vi "ADQ214 Get Afe Switch.vi"(7 "afe":string, 8 "error in (no error)":errorcluster, 9 "channel":u8, 10 "adq214_num":i32, 11 "adq_cu_ptr":u32) -> (0 "error out":errorcluster, 2 "function return":u32, 3 "adq_cu_ptr out":u32, 5 "afe out":string)   [LabVIEW 8.6, in "ADQAPI.lvlib"]
doc: "extern \"C\" __declspec(dllimport) unsigned int ADQ214_GetAfeSwitch(void* adq_cu_ptr, int adq214_num, unsigned char channel, unsigned char* afe);"
uses:
  F/HRT/Sp Devices Thesis/ADQ-214 project (H R)/ADQAPI.lvlib
  F:/HRT/Sp Devices Thesis/ADQ-214 project (H R)/ADQAPI.dll
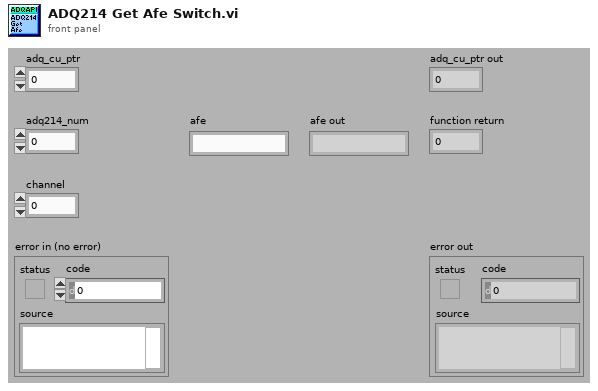
[diagram p1: front panel]
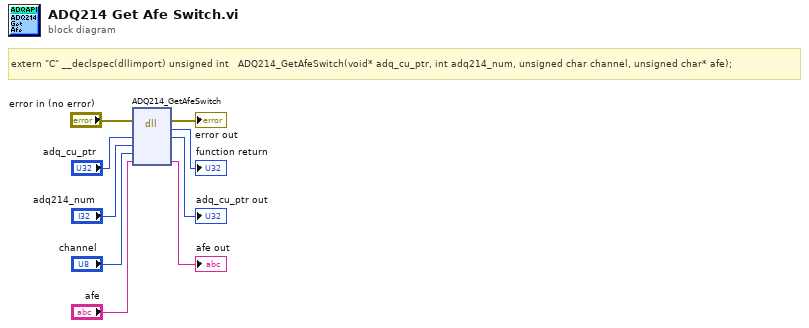
[diagram p0: block diagram]
diagram:
  # "extern \"C\" __declspec(dllimport) unsigned int   ADQ214_GetAfeSwitch(void* adq_cu_ptr, int adq214_num, unsigned char channel, unsigned char* afe);"
  n1 = dll-call lib="F:/HRT/Sp Devices Thesis/ADQ-214 project (H R)/ADQAPI.*" fn="ADQ214_GetAfeSwitch"(error in="error in (no error)", "adq_cu_ptr"="adq_cu_ptr", "adq214_num"="adq214_num", "channel"="channel", "afe"="afe") -> (error out=→"error out":errorcluster, →"function return":u32, "adq_cu_ptr"=→"adq_cu_ptr out":u32, "afe"=→"afe out":string)  [unwired: 4 in, 1 out]
